vi "Add Error.vi"(8 "error in (no error)":errorcluster, 9 "String to Append":string, 10 "Error":T1, 11 "Insert Error":bool=TRUE) -> (0 "error out":errorcluster)   [LabVIEW 2021, in "pcap Parse and Build.lvclass"]
uses:
  pcap Parse and Build.lvclass
  Typedef/Errors.ctl
  <vilib>/CIF Foundation/CIF Utilities/Errors/Errors_CIF_U.lvlib
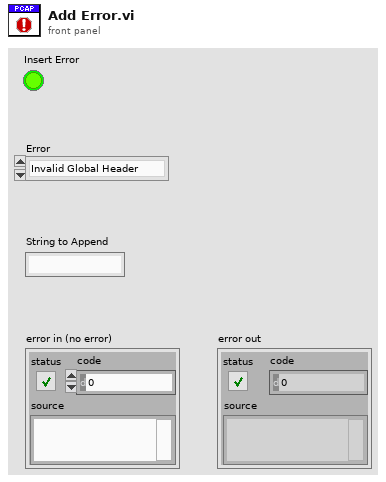
[diagram p1: front panel]
types:
  T1 = typedef "pcap Parse and Build.lvclass/Errors.ctl" = enum16{"Invalid Global Header", "Out of Data"}
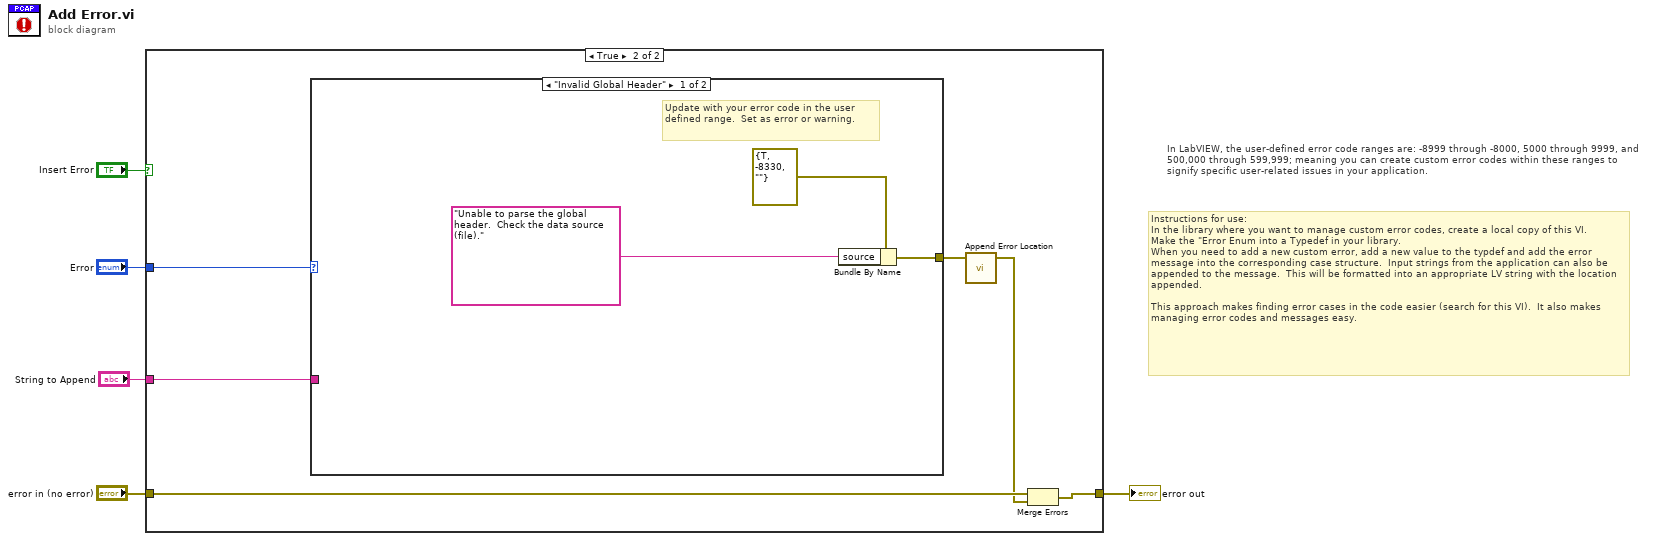
[diagram p0: block diagram]
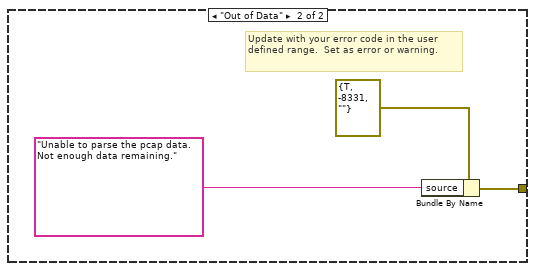
[diagram p3: hidden frame]
diagram:
  # "Instructions for use:\nIn the library where you want to manage custom error codes, create a local copy of this VI.\nMake the \"Error Enum into a Typedef in your library.\nWhen you need to add a new custom error, add a new value to the typdef and add the error message into the corresponding case structure.  Input strings from the application can also be appended to the message.  This will be formatted into an appropriate LV string with the location appended.  \n\nThis approach makes finding error cases in the code easier (search for this VI).  It also makes managing error codes and messages easy."
  # "In LabVIEW, the user-defined error code ranges are: -8999 through -8000, 5000 through 9999, and 500,000 through 599,999; meaning you can create custom error codes within these ranges to signify specific user-related issues in your application."
  n1 = case shown="True" "Insert Error" {
    tunnel: [w6 w9] -> w4
    tunnel: "error in (no error)" -> [w6 w10]
    tunnel: "Error" -> [_ w12]
    tunnel: "String to Append" -> [_ w11]
    frame False {
    }
    frame True {
      n2 = case shown="\"Invalid Global Header\"" w12 {
        tunnel: w11 -> [_ _]
        tunnel: [w14 w17] -> w8
        frame "Invalid Global Header" {
          # "Update with your error code in the user defined range.  Set as error or warning."
          n3 = Bundle By Name(cluster=errorcluster {"status"=TRUE, "code"=-8330, "source"=""} ("Invalid ID"), "source"="Unable to parse the global header.  Check the data source (file).") -> (w14:errorcluster)
        }
        frame "Out of Data" {
          # "Update with your error code in the user defined range.  Set as error or warning."
          n4 = Bundle By Name(cluster=errorcluster {"status"=TRUE, "code"=-8331, "source"=""} ("Invalid ID"), "source"="Unable to parse the pcap data.  Not enough data remaining.") -> (w17:errorcluster)
        }
      }
      n5 = call <vilib>:"Append Error Location.vi"("error in (no error)"=w8) -> ("error out"=w7:errorcluster)  [unwired: 4 in]
      n6 = Merge Errors(w10, w7) -> (w9:errorcluster)
    }
  }
  "error out" <- w4
